vi "BrainTease.vi"() -> ()   [LabVIEW 2018]
uses:
  Interpreter State.ctl
  BrainFuck App Data.ctl
panel:
  out "Script Pointer":u64=12402 format="%#.2p"
  out "State":T1
  in  "Reset":bool
  in  "Run/Pause":bool
  in  "Speed":u16(ring)=250 items=["Fast"=1, "Medium"=100, "Slow"=250]
  out "# Instr":u64=12402 format="%#.2p"
  in  "Cursor":bool
  out "Index":u64=7
  out "Output":string="A"
  in  "Input":string=">>>,.!A"
  in  "Brainfuck Script":string=">>>+[[-]>>[-]++>+>+++++++[<++++>>++<-]++>>+>+>+++++[>++>++++++<<-]+>>>,<++[[>[\n->>]<[>>]<<-]<[<]<+>>[>]>[<+>-[[<+>-]>]<[[[-]<]++<-[<+++++++++>[<->-]>>]>>]]<<\n]<]<[[<]>[[>]>>[>>]+[<<]<[<]<+>>-]>[>]+[->>]<<<<[[<<]<[<]+<<[+>+<<-[>-->+<<-[>\n+<[>>+<<-]]]>[<+>-]<]++>>-->[>]>>[>>]]<<[>>+<[[<]<]>[[<<]<[<]+[-<+>>-[<<+>++>-\n[<->[<<+>>-]]]<[>+<-]>]>[>]>]>[>>]>>]<<[>>+>>+>>]<<[->>>>>>>>]<<[>.>>>>>>>]<<[\n>->>>>>]<<[>,>>>]<<[>+>]<<[+<<]<]\n[input a brainfuck program and its input, separated by an exclamation point.\nDaniel B Cristofani (cristofdathevanetdotcom)\nhttp://www.hevanet.com/cristofd/brainfuck/]"
  out "Pointer":u64=6
  out "Memory U16":u16[](array[numeric])
  # "https://en.wikipedia.org/wiki/Brainfuck"
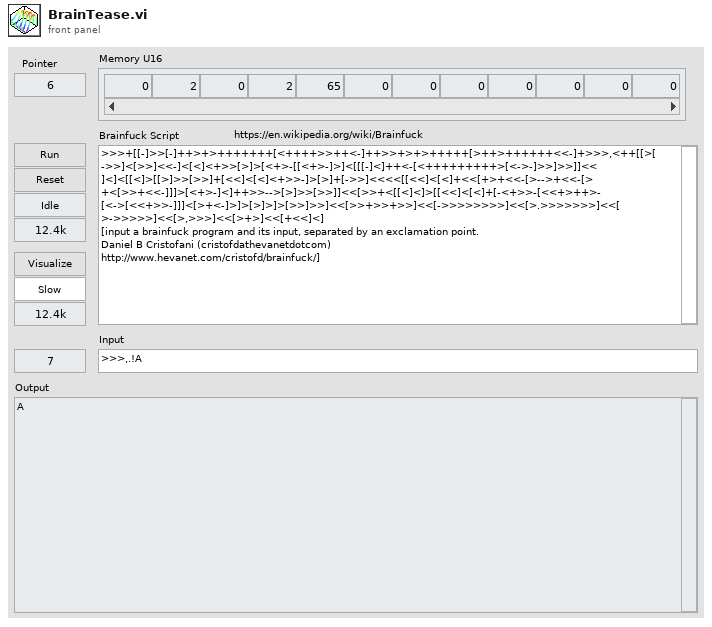
[diagram p1: front panel]
types:
  T1 = typedef "Interpreter State.ctl" = enum16{"Idle", "Init", "Running", "Paused"}
  T2 = typedef "BrainFuck App Data.ctl" = cluster{"Memory":u16[], "Pointer":u64, "Input Pointer":u64, "Script Pointer":u64, "# Instructions":u64, "Output":string, "Input":string, "Bra":u64[], "Ket":u64[], "Script":string, "Length":i32, "Debug":bool}
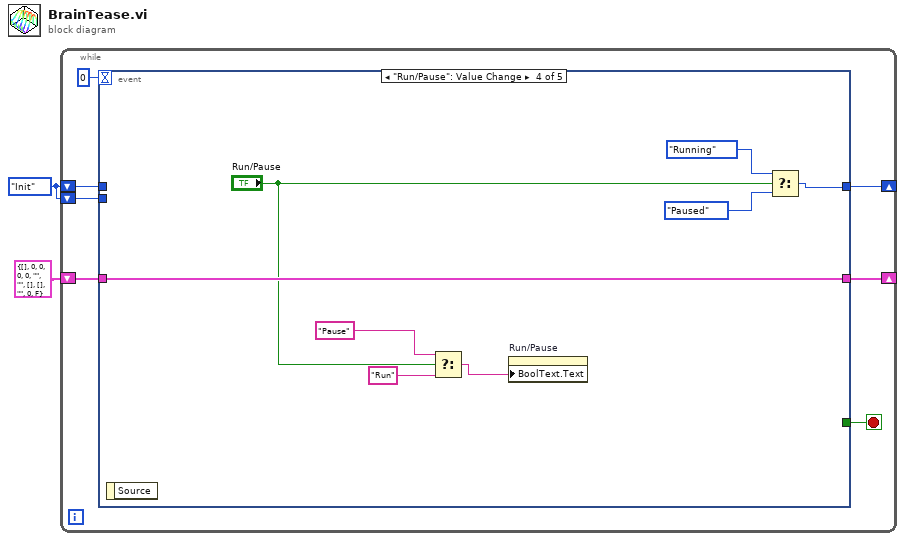
[diagram p0: block diagram]
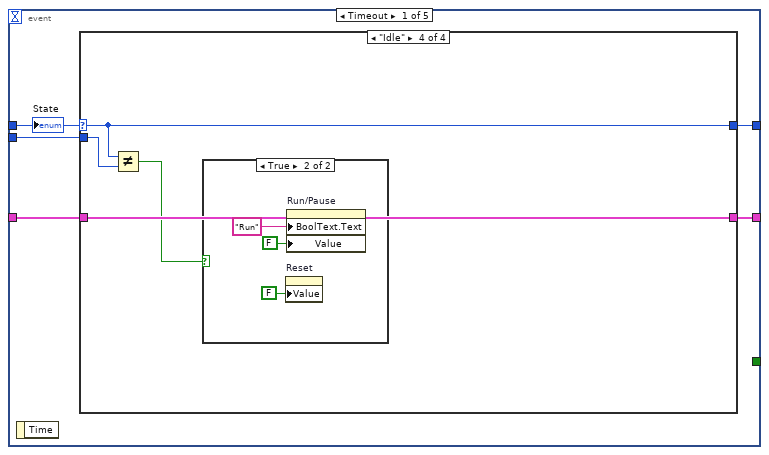
[diagram p2: hidden frame]
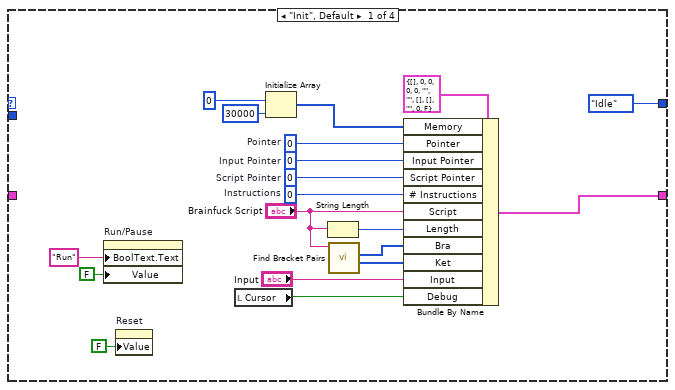
[diagram p3: hidden frame]
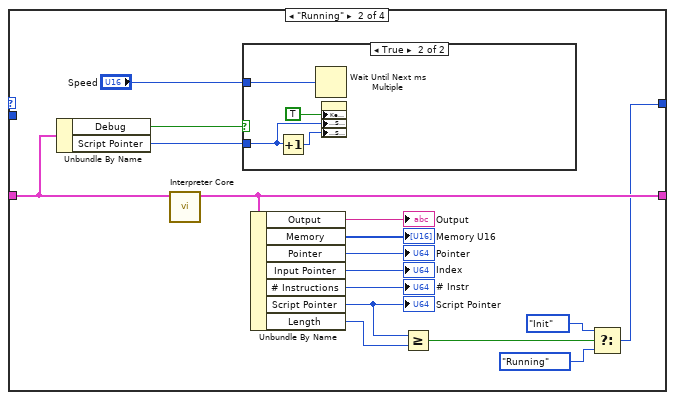
[diagram p4: hidden frame]
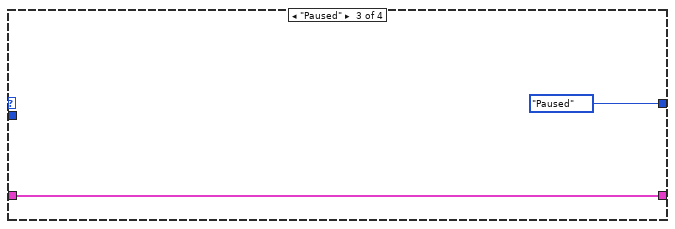
[diagram p6: hidden frame]
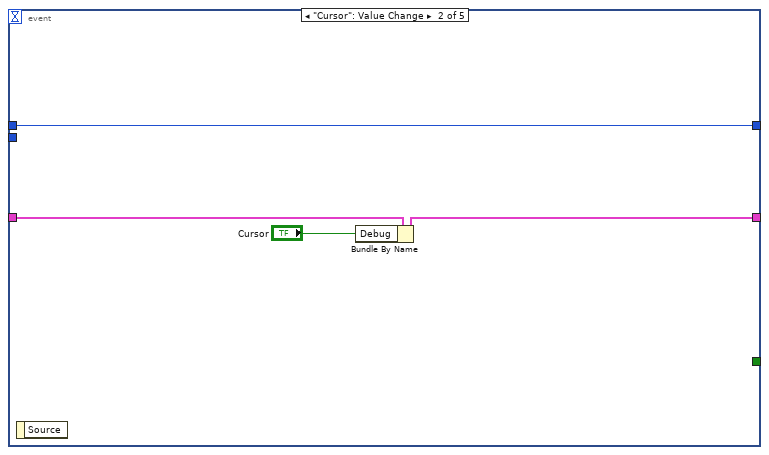
[diagram p8: hidden frame]
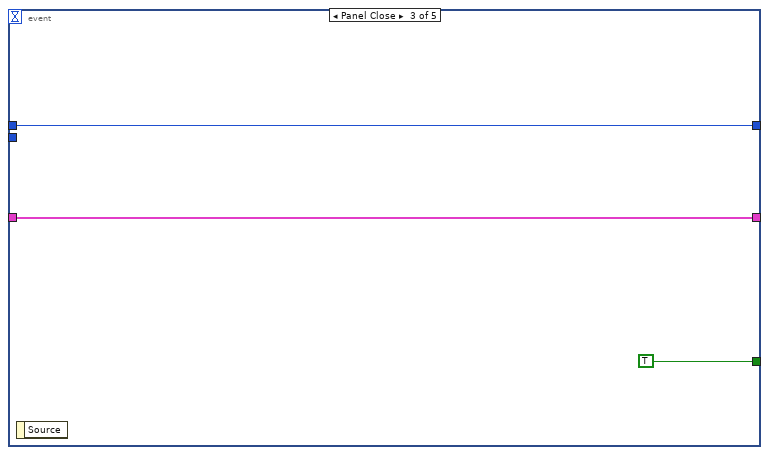
[diagram p9: hidden frame]
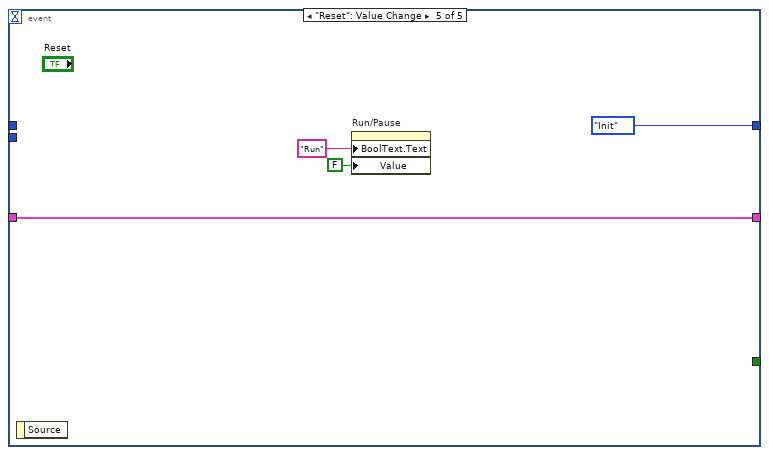
[diagram p10: hidden frame]
diagram:
  w1 = Interpreter_State."Init"
  n1 = while {
    shift-right: [w8] -> _
    shift-left: T2 {"Memory"=[], "Pointer"=0, "Input Pointer"=0, "Script Pointer"=0, "# Instructions"=0, "Output"="", "Input"="", "Bra"=[], "Ket"=[], "Script"="", "Length"=0, "Debug"=FALSE} ("Data Out") -> [w9]
    shift-right: [w4] -> _
    shift-left: w1 -> [w5]
    shift-left: w1 -> [w3]
    stop <- w6 stop-if-true
    n2 = event shown="[3] \"Run/Pause\": Value Change" {
      selector: _ -> [_ _ _ _ _]
      dyn-events: _ -> [_ _ _ _ _]
      timeout: 0 -> [_ _ _ _ _]
      tunnel: w9 -> [w14 w65 w69 w74 w80]
      tunnel: [w13 w64 w69 w74 w80] -> w8
      tunnel: [_ _ TRUE _ _] -> w6
      tunnel: w5 -> [w12 w66 w67 _ _]
      tunnel: [w11 w66 w67 w75 Interpreter_State."Init"] -> w4
      tunnel: w3 -> [w10 _ _ _ _]
      event Timeout {
        n3 = event-data() -> ()  [unwired: 1 in, 1 out]
        n4 = case shown="\"Idle\"" w12 {
          selector: w12 -> [_ _ _ w57]
          tunnel: w14 -> [_ w49 w55 w59]
          tunnel: [w25 w47 w55 w59] -> w13
          tunnel: [Interpreter_State."Idle" w37 Interpreter_State."Paused" w57] -> w11
          tunnel: w10 -> [_ _ _ w58]
          frame "Init", Default {
            w28 = u64 0  # Instructions
            w31 = u64 0  # Pointer
            w29 = u64 0  # Script Pointer
            w30 = u64 0  # Input Pointer
            n5 = property on="Run/Pause" class="Bool (strict)"("BoolText.Text"="Run" ("Boolean Text.Text"), "Value"=FALSE ("Run/Pause")) -> ()  [unwired: 2 in, 2 out]
            n6 = property on="Reset" class="Bool (strict)"("Value"=FALSE ("Reset")) -> ()  [unwired: 2 in, 2 out]
            n7 = local read "Cursor"() -> (w15:bool)
            n8 = Initialize Array(u16 0 ("Memory U8"), 30000 ("dimension size")) -> (w33:u16[])
            n9 = String Length(string="Brainfuck Script") -> (length=w23:i32)
            n10 = call "Find Bracket Pairs.vi"("BrainTease Script"="Brainfuck Script") -> ("Ket"=w20:u64[], "Bra"=w21:u64[])  [unwired: 7 in, 2 out]
            n11 = Bundle By Name(cluster=T2 {"Memory"=[], "Pointer"=0, "Input Pointer"=0, "Script Pointer"=0, "# Instructions"=0, "Output"="", "Input"="", "Bra"=[], "Ket"=[], "Script"="", "Length"=0, "Debug"=FALSE} ("output cluster"), "Memory"=w33, "Pointer"=w31, "Input Pointer"=w30, "Script Pointer"=w29, "# Instructions"=w28, "Script"="Brainfuck Script", "Length"=w23, "Bra"=w21, "Ket"=w20, "Input"="Input", "Debug"=w15) -> (w25:T2)
          }
          frame "Running" {
            n12 = Unbundle By Name(w49) -> ("Debug"=w35:bool, "Script Pointer"=w48:u64)
            n13 = call "Interpreter Core.vi"("Data In"=w49) -> ("Data Out"=w47:T2)  [unwired: 10 in]
            n14 = case shown="True" w35 {
              tunnel: w48 -> [_ w52]
              tunnel: "Speed" -> [_ w50]
              frame False {
              }
              frame True {
                n15 = Increment(x=w52) -> (x+1=w51:u64)
                n16 = Wait Until Next ms Multiple(millisecond multiple=w50) -> ()  [unwired: 1 out]
                n17 = property on="Brainfuck Script" class="Str"("Key Focus"=TRUE, "Text.Selection Start"=w52, "Text.Selection End"=w51) -> ()  [unwired: 2 in, 2 out]
              }
            }
            n18 = Unbundle By Name(w47) -> ("Output"=→"Output":string, "Memory"=→"Memory U16":u16[], "Pointer"=→"Pointer":u64, "Input Pointer"=→"Index":u64, "# Instructions"=→"# Instr":u64, "Script Pointer"=w34:u64, "Length"=w36:i32)
            "Script Pointer" <- w34
            n19 = Greater Or Equal?(x=w34, y=w36) -> (x >= y?=w40:bool)
            n20 = Select(t=Interpreter_State."Init", s=w40, f=Interpreter_State."Running") -> (s? t:f=w37:T1)
          }
          frame "Paused" {
          }
          frame "Idle" {
            n21 = Not Equal?(x=w57, y=w58) -> (x != y?=w56:bool)
            n22 = case shown="True" w56 {
              frame False {
              }
              frame True {
                n23 = property on="Reset" class="Bool (strict)"("Value"=FALSE ("Reset")) -> ()  [unwired: 2 in, 2 out]
                n24 = property on="Run/Pause" class="Bool (strict)"("BoolText.Text"="Run" ("Boolean Text.Text"), "Value"=FALSE ("Run/Pause")) -> ()  [unwired: 2 in, 2 out]
              }
            }
          }
        }
        "State" <- w12
      }
      event "Cursor": Value Change {
        n25 = event-data() -> ()  [unwired: 1 in, 1 out]
        n26 = Bundle By Name(cluster=w65, "Debug"="Cursor") -> (w64:T2)
      }
      event Panel Close {
        n27 = event-data() -> ()  [unwired: 1 in, 1 out]
      }
      event "Run/Pause": Value Change {
        n28 = event-data() -> ()  [unwired: 1 in, 1 out]
        n29 = Select(t="Pause" ("Boolean Text.Text"), s="Run/Pause", f="Run" ("Boolean Text.Text")) -> (s? t:f=w70:string)
        n30 = property on="Run/Pause" class="Bool (strict)"("BoolText.Text"=w70) -> ()  [unwired: 2 in, 2 out]
        n31 = Select(t=Interpreter_State."Running", s="Run/Pause", f=Interpreter_State."Paused") -> (s? t:f=w75:T1)
      }
      event "Reset": Value Change {
        n32 = event-data() -> ()  [unwired: 1 in, 1 out]
        n33 = property on="Run/Pause" class="Bool (strict)"("BoolText.Text"="Run" ("Boolean Text.Text"), "Value"=FALSE ("Run/Pause")) -> ()  [unwired: 2 in, 2 out]
      }
    }
  }
